vi "Dashboard Main.vi"() -> ()   [LabVIEW 2012]
uses:
  <vilib>/event_ctls.llb/eventvkey.ctl
  <vilib>/Utility/config.llb/NI_LVConfig.lvlib
  <vilib>/Utility/config.llb/Read Key (I32).vi
  <vilib>/Utility/config.llb/Write Key (I32).vi
  <vilib>/Rock Robotics/WPI/Camera/WPI_CameraExposure Priority Values.ctl
  <vilib>/Utility/config.llb/Write Key (String).vi
  <vilib>/Utility/config.llb/Read Key (String).vi
  <vilib>/Rock Robotics/WPI/Camera/WPI_CameraWhite Balance Values.ctl
panel:
  out "JS Buttons 1":cluster{bool, bool, bool, bool}={FALSE, TRUE, TRUE, FALSE}
  out "Joystick 2":cluster{"X":dbl, "Y":dbl}[](graph)
  out "Joystick 1":cluster{"X":dbl, "Y":dbl}[](graph)
  in  "STOP":bool
  in  "Camera?":bool
  in  "Brightness":i32=45
  in  "Color Level":i32=90
  in  "White Balance":T1=enum."Hold current"
  in  "Exposure Priority":T2=enum."Prioritize frame rate"
  out "Battery Value":dbl(slide) scale=0.0..14.0 scale format="%#_2e"
  out "Battery":sgl(graph)
  in  "Camera Settings":T3={"Frate Rate"=30, "Compression"=30, "Size"=1} {"Frate Rate" scale=1.0..30.0; "Size" items=["640x480", "320x240", "160x120"]}
  out "Mode":T4(ring)=enum."Auto Disabled"
  out "Robot IP":string
  in  "Dashboard Tab":enum32{"Operation", "Test", "Checklist"}(tab)
  in  "Checkbox 2":bool
  in  "Checkbox 1":bool
  in  "Slider 1":dbl(slide) scale=0.0..100.0
  in  "?":bool
  in  "Slider":dbl(slide) scale=0.0..100.0 scale format="%#_3g"
  in  "On/Off":bool caption="Solenoid"
  in  "Test Name":u16(ring) items=["Select the test to run...", "Example Test", "-------------------------------", "List of tests is built in robot code.", "Replace with your own automated tests."]
  in  "Test Tree":string(tree)
  in  "Motor":cluster{"Value":dbl, "Enable":bool} {"Value" scale=-1.0..1.0 scale format="%#_3g"}
  out "Progress":T5 {"Test Progress" scale=0.0..100.0}
  in  "Rev/Fwd":cluster{"Forward":bool, "Reverse":bool}
  in  "Ring":u16(ring) items=["Auto", "Fixed indoor", "Fixed outdoor 1", "Fixed outdoor 2", "Fixed fluorescent 1", "Fixed fluorescent 2", "Hold current"]
  in  "Listbox":i32(listbox)
  in  "Viewer":enum32{"Camera Image", "Variables"}(tab)
  out "Mbps":dbl format="%#.1g"
  in  "Enable":bool
  in  "DB Camera Config":bool
  out "Mbps":bool
  out "fps":dbl format="%#.1g"
  out "Image Error Message":string="Timeout in Camera Communications"
  out "Camera Image":T6(plugin-control)
  out "Tree":string(tree)
  # "Drive & Motors"
  # "Robot IP:"
  # "Customize by placing controls and indicators here and name to match\nDashboard Variables on robot."
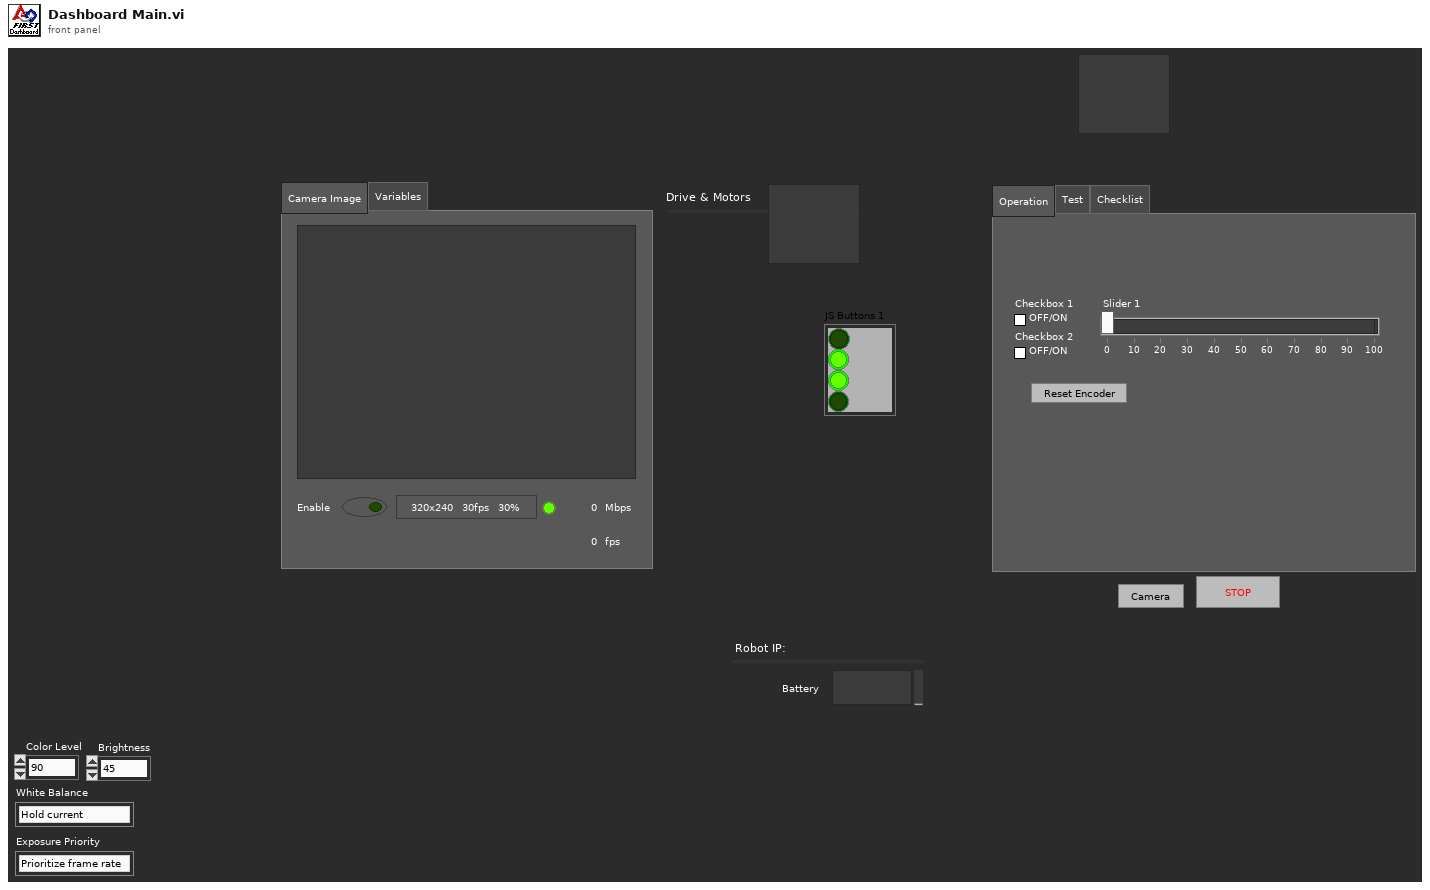
[diagram p1: front panel]
types:
  T1 = typedef "WPI_CameraWhite Balance Values.ctl" = enum16{"Auto", "Fixed indoor", "Fixed outdoor 1", "Fixed outdoor 2", "Fixed fluorescent 1", "Fixed fluorescent 2", "Hold current"}
  T2 = typedef "WPI_CameraExposure Priority Values.ctl" = enum16{"None", "Prioritize frame rate", "Prioritize image quality"}
  T3 = cluster{"Frate Rate":i32, "Compression":i32, "Size":u16}
  T4 = enum8{"Tele-Op Disabled", "Tele-Op Enabled", "Auto Disabled", "Auto Enabled", "Test Disabled", "Test Enabled", ""}
  T5 = cluster{"Test Progress":u8, "Test Progress Text":string}
  T6 = typedef "IMAQ Image.ctl" = refnum<image>
  T7 = typedef "Image Type" = u32
  T8 = cluster{"Left":i32, "Top":i32, "Right":i32, "Bottom":i32}
  T9 = typedef "WPI_CameraDevRef.ctl" = cluster{"Camera Address":string, "CameraStatus":errorcluster, "Acquire Image Notifier":refnum<notifier>}
  T10 = typedef "LVRectTypeDef.ctl" = cluster{"Left":i16, "Top":i16, "Right":i16, "Bottom":i16}
  T11 = cluster{"Competition mode":bool, "Robot Link":bool, "Autonomous":bool, "Enabled":bool, "E-Stop":bool, "Simulated":bool, "TestMode":bool, "Docked Window":bool}
  T12 = typedef "NI_LVConfig.lvlib/Config Data RefNum.ctl" = refnum<k1>
  T13 = typedef "eventvkey.ctl" = enum16{"ASCII", "Enter", "Return", "Shift", "Ctrl", "Alt", "Cmd", "Opt", "Caps", "NumLock", "Clear", "Break", "Up", "Down", "Left", "Right", "Insert", "Delete", "Home", "End", "PageUp", "PageDown", "Escape", "Help", "Pause", "ScrollLock", "F1", "F2", "F3", "F4", "F5", "F6", "F7", "F8", "F9", "F10", "F11", "F12", "F13", "F14", "F15", "F16", "F17", "F18", "F19", "F20", "F21", "F22", "F23", "F24", "Play", "VolumeUp", "VolumeDown", "Mute", "Two Byte Char"}
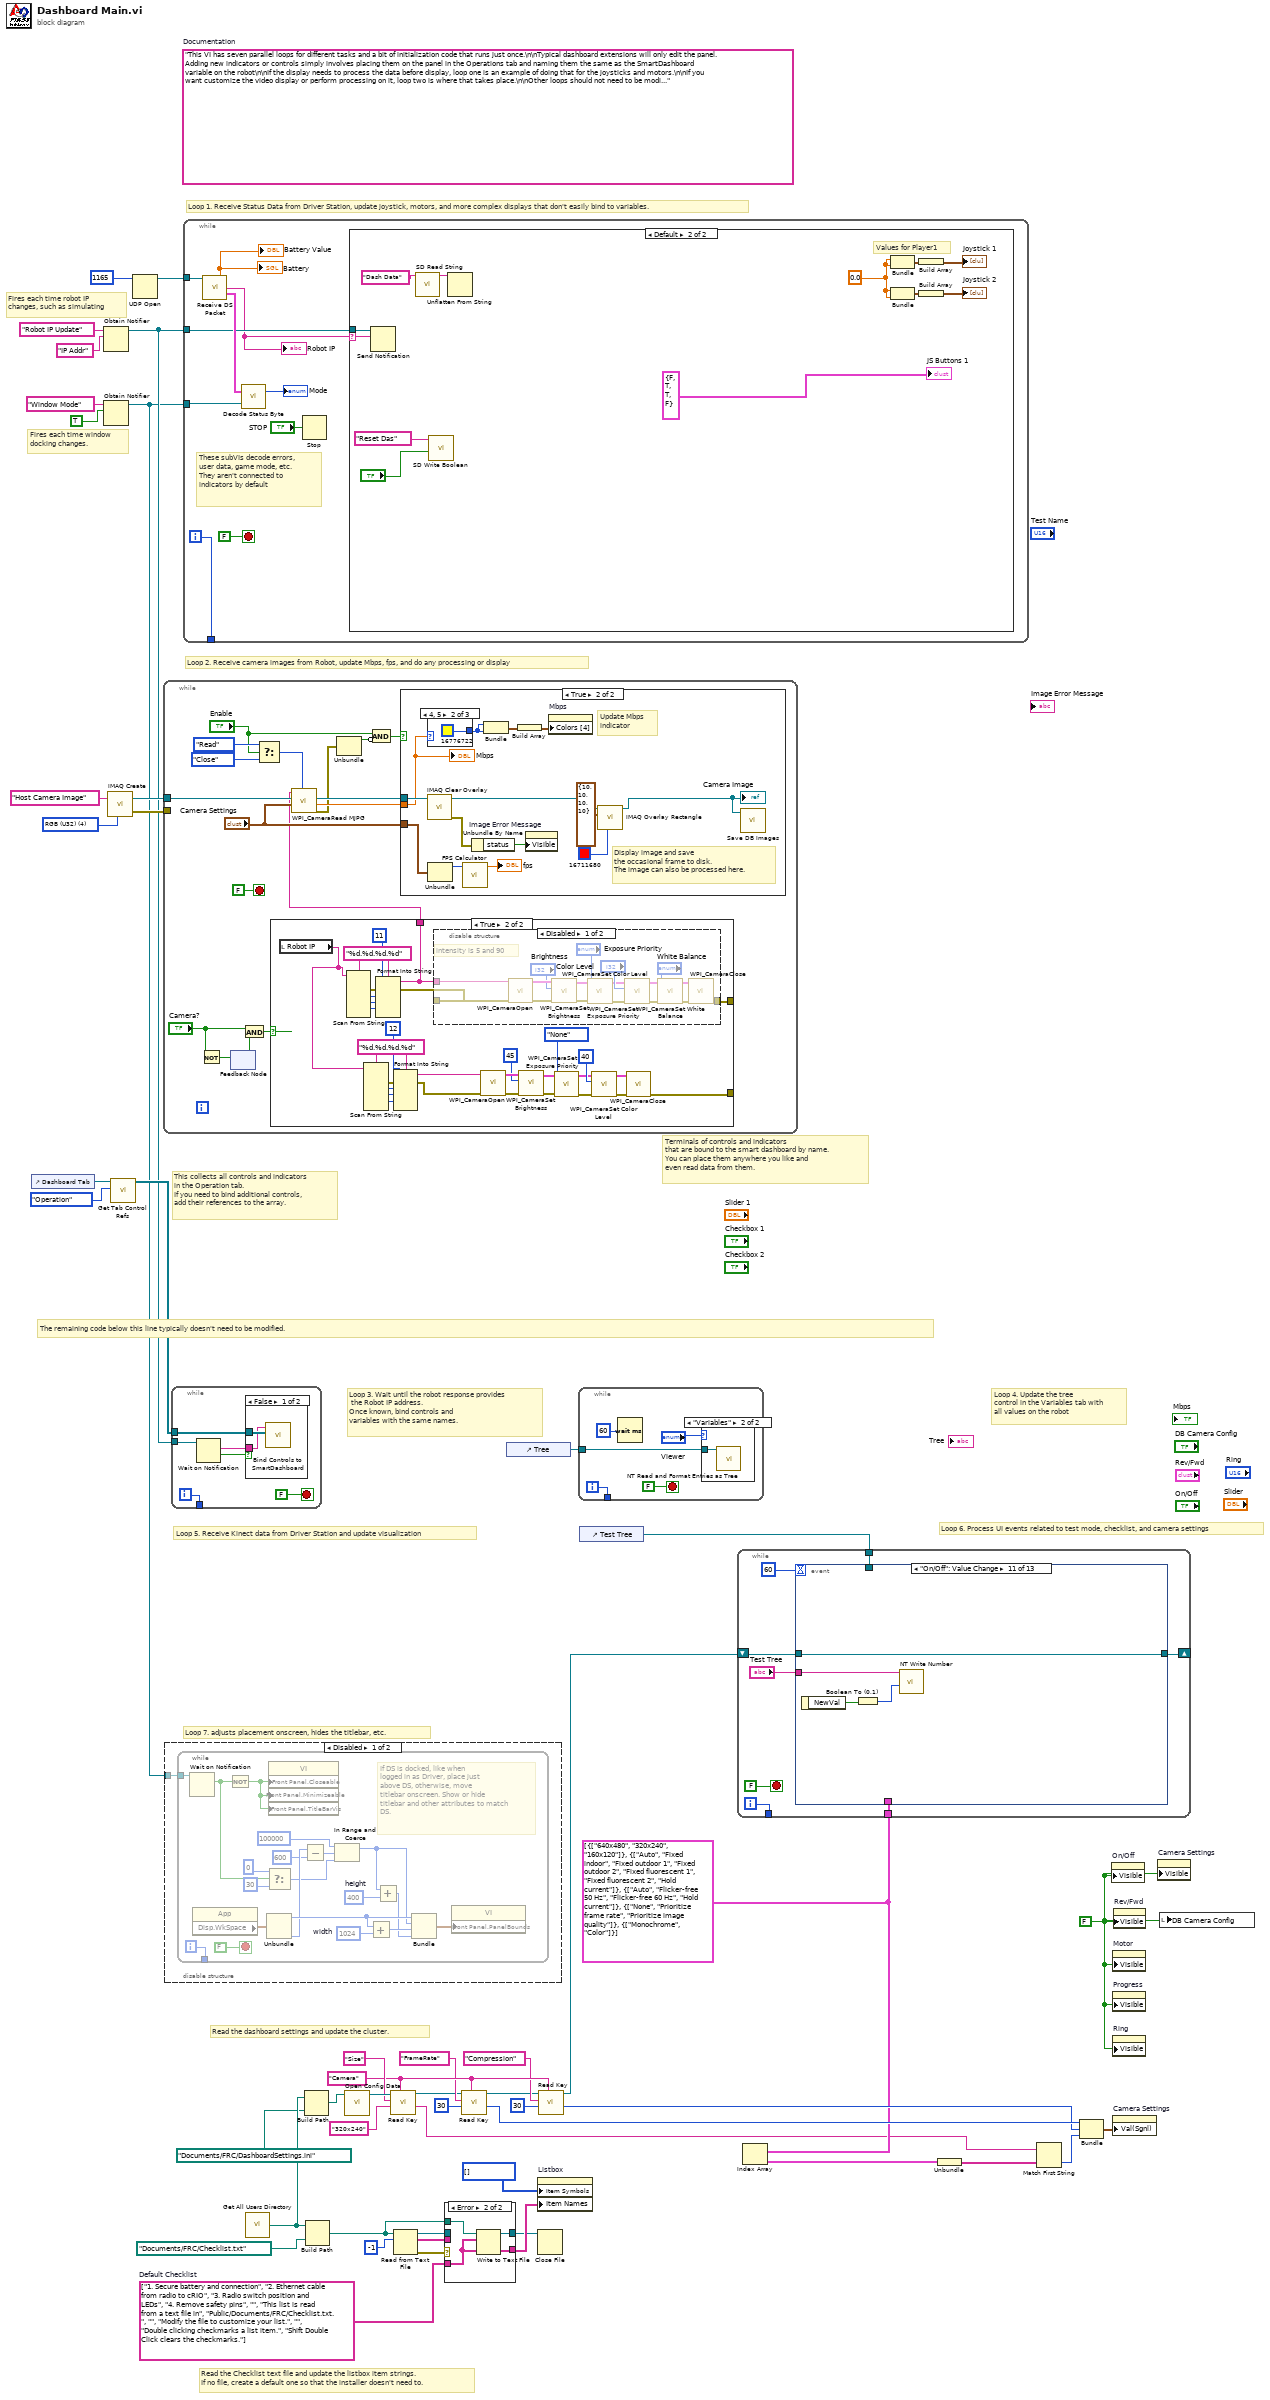
[diagram p0: block diagram]
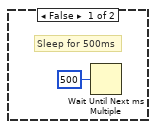
[diagram p6: hidden frame]
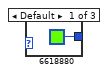
[diagram p7: hidden frame]
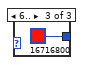
[diagram p8: hidden frame]
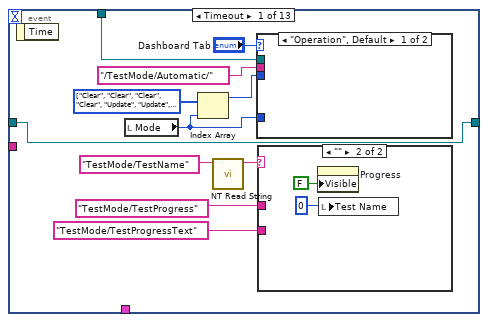
[diagram p10: hidden frame]
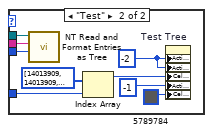
[diagram p11: hidden frame]
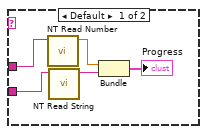
[diagram p12: hidden frame]
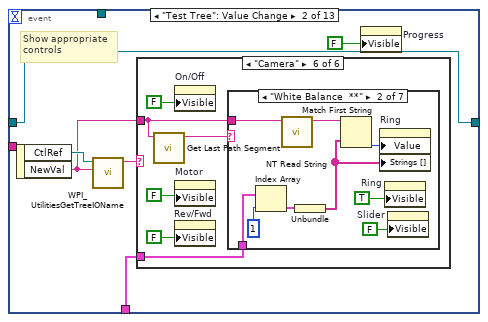
[diagram p13: hidden frame]
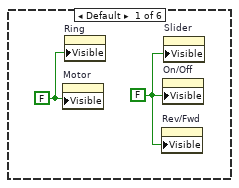
[diagram p14: hidden frame]
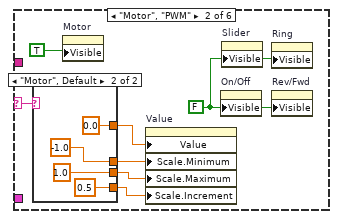
[diagram p15: hidden frame]
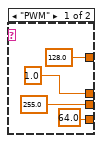
[diagram p16: hidden frame]
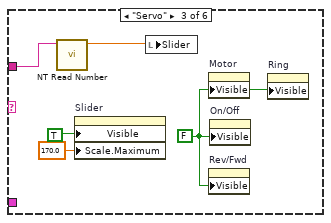
[diagram p17: hidden frame]
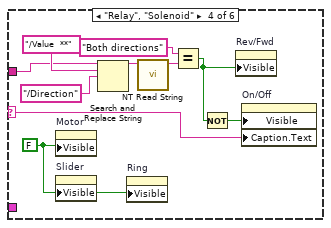
[diagram p18: hidden frame]
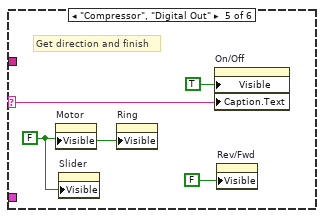
[diagram p19: hidden frame]
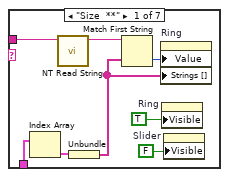
[diagram p20: hidden frame]
diagram:
  w21 = "Camera"
  w13 = cluster{string[]}[] [{["640x480", "320x240", "160x120"]}, {["Auto", "Fixed indoor", "Fixed outdoor 1", "Fixed outdoor 2", "Fixed fluorescent 1", "Fixed fluorescent 2", "Hold current"]}, {["Auto", "Flicker-free 50 Hz", "Flicker-free 60 Hz", "Hold current"]}, {["None", "Prioritize frame rate", "Prioritize image quality"]}, {["Monochrome", "Color"]}]
  w29 = string[] ["1. Secure battery and connection", "2. Ethernet cable from radio to cRIO", "3. Radio switch position and LEDs", "4. Remove safety pins", "", "This list is read from a text file in", "Public/Documents/FRC/Checklist.txt.", "", "Modify the file to customize your list.", "", "Double clicking checkmarks a list item.", "Shift Double Click clears the checkmarks."]  # Default Checklist
  w27 = FALSE ("Visible")
  (unwired) "This VI has seven parallel loops for different tasks and a bit of initialization code that runs just once.\n\nTypical dashboard extensions will only edit the panel. Adding new indicators or controls simply involves placing them on the panel in the Operations tab and naming them the same as the SmartDashboard variable on the robot\n\nIf the display needs to process the data before display, loop one is an example of doing that for the joysticks and motors.\n\nIf you want customize the video display or perform processing on it, loop two is where that takes place.\n\nOther loops should not need to be modified. They are pretty standard, and document the task they perform."  # Documentation
  w48 = T7 4 items=["Grayscale (U8)", "Grayscale (I16)", "Grayscale (SGL)", "Complex (CSG)", "RGB (U32)", "HSL (U32)", "RGB (U64)"] ("Image Type")
  # "Fires each time robot IP\nchanges, such as simulating"
  # "Fires each time window\ndocking changes."
  # "Read the Checklist text file and update the listbox item strings.\nIf no file, create a default one so that the installer doesn't need to."
  # "This collects all controls and indicators\nin the Operation tab.\nIf you need to bind additional controls,\nadd their references to the array."
  # "The remaining code below this line typically doesn't need to be modified."
  # "Loop 6. Process UI events related to test mode, checklist, and camera settings"
  # "Read the dashboard settings and update the cluster."
  # "Terminals of controls and indicators\nthat are bound to the smart dashboard by name.\nYou can place them anywhere you like and\neven read data from them."
  # "Loop 4. Update the tree\ncontrol in the Variables tab with\nall values on the robot"
  # "Loop 3. Wait until the robot response provides\n the Robot IP address.\nOnce known, bind controls and\nvariables with the same names."
  # "Loop 5. Receive Kinect data from Driver Station and update visualization"
  # "Loop 7. adjusts placement onscreen, hides the titlebar, etc."
  # "Loop 1. Receive Status Data from Driver Station, update joystick, motors, and more complex displays that don't easily bind to variables."
  # "Loop 2. Receive camera images from Robot, update Mbps, fps, and do any processing or display"
  n1 = control-ref of="Dashboard Tab"() -> (w43:refnum<vi>)
  n2 = Obtain Notifier(name (unnamed)="Robot IP Update", notification data type="IP Addr" ("name (unnamed)")) -> (notifier out=w40:refnum<notifier>)  [unwired: 2 in, 2 out]
  n3 = Obtain Notifier(name (unnamed)="Window Mode", notification data type=TRUE) -> (notifier out=w33:refnum<notifier>)  [unwired: 2 in, 2 out]
  n4 = call "IMAQ Create"("Image Name"="Host Camera Image", "Image Type"=w48) -> ("New Image"=w46:T6, "error out"=w45:errorcluster)  [unwired: 2 in, 1 out]
  n5 = call <vilib>:"Get Tab Control Refs.vi"("Page Index"=enum32{"Operation", "Test"}."Operation" ("Dashboard Tab"), "TabControl in"=w43) -> ("ControlsOnPage"=w44:refnum<vi>[])  [unwired: 9 in]
  n6 = UDP Open(11:u16 1165 ("port")) -> (port=w49:refnum<k16>)  [unwired: 2 in, 4 out]
  n7 = while {
    tunnel: w46 -> [w65]
    tunnel: w45 -> [_]
    stop <- FALSE stop-if-true
    n8 = Not(x="Camera?") -> (.not. x?=w55:bool)
    n9 = feedback #1() -> (w54:bool)  [unwired: 1 in]
    n10 = feedback-in #1(w55) -> ()
    n11 = And(x="Camera?", y=w54) -> (x .and. y?=w52:bool)
    n12 = Select(t=enum16{"Read", "Reopen", "Close"}."Read" ("Operation"), s="Enable", f=enum16{"Read", "Reopen", "Close"}."Close" ("Operation")) -> (s? t:f=w60:enum16{"Read", "Reopen", "Close"})
    n13 = case shown="True" w52 {
      tunnel: [_ w90] -> _
      tunnel: [_ w70] -> _
      tunnel: [_ w68] -> w51
      frame False {
      }
      frame True {
        w77 = "%d.%d.%d.%d" ("format string")
        w92 = "%d.%d.%d.%d" ("format string")
        n14 = local read "Robot IP"() -> (w69:string)
        n15 = Scan From String(format string=w92, input string=w69) -> (error out=w94:errorcluster, output 1=w95:i32, output 2=w96:i32, output 3=w97:i32)  [unwired: 2 in, 7 out]
        n16 = Scan From String(format string=w77, input string=w69) -> (error out=w79:errorcluster, output 1=w80:i32, output 2=w81:i32, output 3=w82:i32)  [unwired: 2 in, 7 out]
        n17 = Format Into String(format string=w92, error in=w94, w95, w96, w97, 11 ("IP Suffix:")) -> (resulting string=w68:string, error out=w91:errorcluster)  [unwired: 1 in]
        n18 = Format Into String(format string=w77, error in=w79, w80, w81, w82, 12 ("IP Suffix:")) -> (resulting string=w71:string, error out=w72:errorcluster)  [unwired: 1 in]
        n19 = disable-structure shown="Disabled" {
          disable-tunnel: w91 -> [w106 _]
          disable-tunnel: w68 -> [w105 _]
          disable-tunnel: [w104 _] -> w90
          frame Disabled {
            # "intensity is 5 and 90"
            n20 = call <vilib>:"WPI_CameraOpen.vi"("error in (no error)"=w106, "Camera Address"=w105) -> ("error out"=w109:errorcluster, "CameraDevRef"=w111:T9)  [unwired: 8 in]
            n21 = call <vilib>:"WPI_CameraSet Brightness.vi"("error in (no error)"=w109, "Brightness"="Brightness", "CameraDevRef"=w111) -> ("error out"=w108:errorcluster, "CameraDevRef Out"=w98:T9)  [unwired: 7 in]
            n22 = call <vilib>:"WPI_CameraSet Exposure Priority.vi"("error in (no error)"=w108, "Exposure Priority"="Exposure Priority", "CameraDevRef"=w98) -> ("error out"=w107:errorcluster, "CameraDevRef Out"=w113:T9)  [unwired: 7 in]
            n23 = call <vilib>:"WPI_CameraSet Color Level.vi"("error in (no error)"=w107, "Color Level"="Color Level", "CameraDevRef"=w113) -> ("error out"=w100:errorcluster, "CameraDevRef Out"=w101:T9)  [unwired: 7 in]
            n24 = call <vilib>:"WPI_CameraSet White Balance.vi"("error in (no error)"=w100, "White Balance"="White Balance", "CameraDevRef"=w101) -> ("error out"=w99:errorcluster, "CameraDevRef Out"=w102:T9)  [unwired: 7 in]
            n25 = call <vilib>:"WPI_CameraClose.vi"("error in (no error)"=w99, "CameraDevRef"=w102) -> ("error out"=w104:errorcluster)  [unwired: 9 in]
          }
          frame Enabled {
          }
        }
        n26 = call <vilib>:"WPI_CameraOpen.vi"("error in (no error)"=w72, "Camera Address"=w71) -> ("error out"=w76:errorcluster, "CameraDevRef"=w84:T9)  [unwired: 8 in]
        n27 = call <vilib>:"WPI_CameraSet Brightness.vi"("error in (no error)"=w76, "Brightness"=45, "CameraDevRef"=w84) -> ("error out"=w75:errorcluster, "CameraDevRef Out"=w85:T9)  [unwired: 7 in]
        n28 = call <vilib>:"WPI_CameraSet Exposure Priority.vi"("error in (no error)"=w75, "Exposure Priority"=WPI_CameraExposure_Priority_Values."None", "CameraDevRef"=w85) -> ("error out"=w74:errorcluster, "CameraDevRef Out"=w88:T9)  [unwired: 7 in]
        n29 = call <vilib>:"WPI_CameraSet Color Level.vi"("error in (no error)"=w74, "Color Level"=40, "CameraDevRef"=w88) -> ("error out"=w73:errorcluster, "CameraDevRef Out"=w87:T9)  [unwired: 7 in]
        n30 = call <vilib>:"WPI_CameraClose.vi"("error in (no error)"=w73, "CameraDevRef"=w87) -> ("error out"=w70:errorcluster)  [unwired: 9 in]
      }
    }
    n31 = call <vilib>:"WPI_CameraRead MJPG.vi"("Operation"=w60, "Camera Settings"="Camera Settings", "Image"=w65, "address"=w51) -> ("error out"=w59:errorcluster, "Bandwidth (kbps)"=w63:dbl, "Image Out"=w64:T6)  [unwired: 5 in]
    n32 = Unbundle(w59) -> ("status"=w57:bool)  [unwired: 2 out]
    n33 = Compound Arithmetic op=AND("Enable", invert w57) -> (w56:bool)
    n34 = case shown="True" w56 {
      tunnel: "Camera Settings" -> [_ w121]
      tunnel: w64 -> [_ w124]
      tunnel: w63 -> [_ w123]
      frame False {
        # "Sleep for 500ms"
        n35 = Wait Until Next ms Multiple(millisecond multiple=u32 500) -> ()  [unwired: 1 out]
      }
      frame True {
        # "Display image and save\nthe occasional frame to disk.\nThe image can also be processed here."
        # "Update Mbps\nindicator"
        n36 = call "IMAQ Clear Overlay"("Image"=w124) -> ("error out"=w128:errorcluster, "Image Out"=w119:T6)  [unwired: 2 in, 7 out]
        n37 = case shown="4, 5" w123 {
          tunnel: [u32 6618880 ("Color Box") u32 16776722 ("Color Box") u32 16716800 ("Color Box")] -> w125
          frame Default {
          }
          frame 4, 5 {
          }
          frame 6.. {
          }
        }
        n38 = Unbundle(w121) -> ("Frate Rate"=w120:i32)  [unwired: 2 out]
        n39 = call "FPS Calculator.vi"("Average Count"=w120) -> ("fps"=→"fps":dbl)  [unwired: 10 in]
        n40 = Unbundle By Name(w128) -> ("status"=w129:bool)
        n41 = Bundle("Color Box"=w125, "Color Box"=w125) -> (w127:cluster{"Color Box":u32, "Color Box":u32})  [unwired: 1 out]
        n42 = Build Array(w127) -> (w126:cluster{"Color Box":u32, "Color Box":u32}[])
        n43 = property on="Image Error Message" class="Str"("Visible"=w129) -> ()  [unwired: 2 in, 2 out]
        n44 = property on="Mbps" class="Bool (strict)"("Colors [4]"=w126) -> ()  [unwired: 2 in, 2 out]
        n45 = call "IMAQ Overlay Rectangle"("Color"=u32 16711680, "Rectangle"=T8 {"Left"=10, "Top"=10, "Right"=10, "Bottom"=10}, "Image"=w119) -> ("Image Out"=w118:T6)  [unwired: 7 in, 1 out]
        "Camera Image" <- w118
        n46 = call "Save DB Images.vi"("Image"=w118) -> ()  [unwired: 2 in, 1 out]
        "Mbps" <- w123
      }
    }
  }
  n47 = disable-structure shown="Disabled" {
    disable-tunnel: w33 -> [w133 _]
    frame Disabled {
      n48 = while {
        tunnel: w133 -> [w152]
        tunnel: [w150] -> _
        i -> [w150]
        stop <- FALSE stop-if-true
        w142 = 1024  # width
        w145 = 400  # height
        # "If DS is docked, like when\nlogged in as Driver, place just\nabove DS, otherwise, move\ntitlebar onscreen. Show or hide\ntitlebar and other attributes to match\nDS."
        n49 = Wait on Notification(notifier=w152) -> (notification=w137:bool)  [unwired: 3 in, 3 out]
        n50 = property class="App"() -> ("Disp.WkSpace"=w148:T10)  [unwired: 2 in, 2 out]
        n51 = Not(x=w137) -> (.not. x?=w151:bool)
        n52 = Unbundle(w148) -> ("Left"=w146:i16, "Bottom"=w143:i16)  [unwired: 2 out]
        n53 = Select(t=0, s=w137, f=30) -> (s? t:f=w136:i32)
        n54 = property class="VI"("Front Panel.Closeable"=w151, "Front Panel.Minimizeable"=w151, "Front Panel.TitleBarVis"=w151) -> ()  [unwired: 2 in, 2 out]
        n55 = Subtract(x=w143, y=600) -> (x-y=w140:i32)
        n56 = In Range and Coerce(upper limit=100000, x=w140, lower limit=w136) -> (coerced(x)=w134:i32)  [unwired: 1 out]
        n57 = Add(x=w146, y=w142) -> (x+y=w147:i32)
        n58 = Add(x=w134, y=w145) -> (x+y=w144:i32)
        n59 = Bundle("Left"=w146, w134, w147, w144) -> (w149:cluster{"Left":i16, i32, i32, i32})  [unwired: 1 out]
        n60 = property class="VI"("Front Panel.PanelBounds"=w149) -> ()  [unwired: 2 in, 2 out]
      }
    }
    frame Enabled {
    }
  }
  n61 = while {
    tunnel: w44 -> [w159]
    tunnel: w40 -> [w156]
    tunnel: [w154] -> _
    i -> [w154]
    stop <- FALSE stop-if-true
    n62 = Wait on Notification(notifier=w156) -> (notification=w155:string, timed out?=w157:bool)  [unwired: 3 in, 2 out]
    n63 = case shown="False" w157 {
      tunnel: w159 -> [w161 _]
      tunnel: w155 -> [w160 _]
      frame False {
        n64 = call <vilib>:"Bind Controls to SmartDashboard.vi"("Bound Control Refs"=w161, "Server IP Address"=w160) -> ()  [unwired: 10 in]
      }
      frame True {
      }
    }
  }
  n65 = while {
    tunnel: w49 -> [w169]
    tunnel: w40 -> [w164]
    tunnel: w33 -> [w167]
    tunnel: [w165] -> _
    i -> [w165]
    stop <- FALSE stop-if-true
    # "These subVIs decode errors, user data, game mode, etc.\nThey aren't connected to indicators by default"
    n66 = call "Receive DS Packet.vi"("Recv Socket"=w169) -> ("Battery"=→"Battery" →"Battery Value":sgl, "Robot IP Address"=w163:string, "Status"=w170:T11)  [unwired: 1 in, 11 out]
    "Robot IP" <- w163
    n67 = call "Decode Status Byte.vi"("Window Mode Notifier"=w167, "Status"=w170) -> ("Mode"=→"Mode":T4)  [unwired: 1 out]
    n68 = Stop(stop? (T)="STOP") -> ()
    n69 = case shown="Default" w163 {
      selector: w163 -> [_ w182]
      tunnel: w164 -> [_ w183]
      frame "0.0.0.0" {
        # "Robot not responding, don't poll the variables"
      }
      frame Default {
        w173 = 0.0
        # "Values for Player1"
        n70 = Send Notification(notification=w182, notifier=w183) -> ()  [unwired: 1 in, 2 out]
        n71 = call <vilib>:"SD Read String.vi"("Name"="Dash Data") -> ("String"=w180:string)  [unwired: 8 in, 2 out]
        n72 = call <vilib>:"SD Write Boolean.vi"("Boolean"="?", "Name"="Reset Das") -> ()  [unwired: 8 in, 2 out]
        n73 = Unflatten From String(binary string=w180) -> ()  [unwired: 4 in, 3 out]
        n74 = Bundle(w173, w173) -> (w177:cluster{dbl, dbl})  [unwired: 1 in]
        n75 = Bundle(w173, w173) -> (w175:cluster{dbl, dbl})  [unwired: 1 in]
        n76 = Build Array(w177) -> (→"Joystick 1":cluster{dbl, dbl}[])
        n77 = Build Array(w175) -> (→"Joystick 2":cluster{dbl, dbl}[])
        "JS Buttons 1" <- cluster{bool, bool, bool, bool} {FALSE, TRUE, TRUE, FALSE} ("JS Buttons 1")
      }
    }
  }
  n78 = call "Get All Users Directory.vi"() -> ("All User Path"=w26:path)
  n79 = Build Path(base path=w26, name or relative path=path "Documents/FRC/DashboardSettings.ini") -> (appended path=w25:path)
  n80 = Build Path(base path=w26, name or relative path=path "Documents/FRC/Checklist.txt") -> (appended path=w30:path)
  n81 = call <vilib>:"Open Config Data.vi"("configuration file path"=w25) -> ("refnum"=w24:T12)  [unwired: 8 in, 2 out]
  n82 = call-poly <vilib>:"Read Key.vi"("section"=w21, "default value"="320x240", "key"="Size", "refnum"=w24) -> ("value"=w11:string, "refnum out"=w6:T12)  [unwired: 2 in, 4 out]
  n83 = Read from Text File(file (use dialog)=w30, count=-1 ("timeout ms (25000)")) -> (refnum out=w8:refnum<file>, text=w31:string[], error out=w32:errorcluster)  [unwired: 2 in, 1 out]
  n84 = case shown="Error" w32 {
    tunnel: w31 -> [w185 _]
    tunnel: [w185 w187] -> w28
    tunnel: w29 -> [_ w187]
    tunnel: w30 -> [_ w188]
    tunnel: [w184 w186] -> w7
    tunnel: w8 -> [w184 _]
    frame No Error {
    }
    frame Error {
      n85 = Write to Text File(file (use dialog)=w188, text=w187) -> (refnum out=w186:refnum<file>)  [unwired: 2 in, 2 out]
    }
  }
  n86 = call-poly <vilib>:"Read Key.vi"("section"=w21, "default value"=30, "key"="FrameRate", "refnum"=w6) -> ("value"=w16:i32, "refnum out"=w5:T12)  [unwired: 1 in, 5 out]
  n87 = control-ref of="Tree"() -> (w2:refnum<vi>)
  n88 = property on="Listbox" class="LstBox (strict)"("Item Symbols"=i32[] [], "Item Names"=w28) -> ()  [unwired: 2 in, 2 out]
  n89 = Close File(refnum=w7) -> ()  [unwired: 1 in, 2 out]
  n90 = call-poly <vilib>:"Read Key.vi"("section"=w21, "default value"=30, "key"="Compression", "refnum"=w5) -> ("value"=w15:i32, "refnum out"=w3:T12)  [unwired: 1 in, 5 out]
  n91 = while {
    tunnel: [w190] -> _
    tunnel: w2 -> [w189]
    i -> [w190]
    stop <- FALSE stop-if-true
    n92 = Wait (ms)(milliseconds to wait=u32 60) -> ()  [unwired: 1 out]
    n93 = case shown="\"Variables\"" "Viewer" {
      tunnel: w189 -> [_ w194]
      frame Default {
      }
      frame "Variables" {
        n94 = call <vilib>:"NT Read and Format Entries as Tree.vi"("Tree Refnum"=w194) -> ()  [unwired: 9 in, 2 out]
      }
    }
  }
  n95 = control-ref of="Test Tree"() -> (w1:refnum<vi>)
  n96 = while {
    tunnel: w13 -> [w199]
    shift-right: [w198] -> _
    shift-left: w3 -> [w197]
    tunnel: [w196] -> _
    tunnel: w1 -> [w195]
    i -> [w196]
    stop <- FALSE stop-if-true
    n97 = event shown="[10] \"On/Off \": Value Change" {
      selector: _ -> [_ _ _ _ _ _ _ _ _ _ _ _ _]
      dyn-events: _ -> [_ _ _ _ _ _ _ _ _ _ _ _ _]
      timeout: u32 60 ("milliseconds to wait") -> [_ _ _ _ _ _ _ _ _ _ _ _ _]
      tunnel: w195 -> [w209 _ _ _ _ _ _ _ _ _ _ _ _]
      tunnel: "Test Tree" -> [_ _ _ _ _ _ _ _ w403 w411 w413 w417 w425]
      tunnel: w199 -> [_ w231 _ _ _ _ w367 w397 _ _ _ _ _]
      tunnel: [w203 w230 _ w333 w341 w353 w366 w390 w402 w409 w412 w416 w424] -> w198
      tunnel: w197 -> [w203 w230 _ w333 w341 w353 w365 w390 w402 w409 w412 w416 w424]
      event Timeout {
        w208 = enum16{"Update", "Clear"}[] [enum."Clear", enum."Clear", enum."Clear", enum."Clear", enum."Update", enum."Update", enum."Clear"] items=["Update", "Clear"]
        n98 = event-data() -> ()  [unwired: 1 in, 1 out]
        n99 = local read "Mode"() -> (w206:T4)
        n100 = Index Array(array=w208, index=w206) -> (element=w207:enum16{"Update", "Clear"})
        n101 = call <vilib>:"NT Read String.vi"("Name"="TestMode/TestName") -> ("String"=w212:string)  [unwired: 9 in, 1 out]
        n102 = case shown="\"Operation\", Default" "Dashboard Tab" {
          tunnel: w209 -> [_ w222]
          tunnel: "/TestMode/Automatic/" ("Name Pattern") -> [_ w221]
          tunnel: w207 -> [_ w220]
          tunnel: w206 -> [_ w218]
          frame "Operation", Default {
          }
          frame "Test" {
            w217 = -2 ("Active Item:Row Number")
            n103 = call <vilib>:"NT Read and Format Entries as Tree.vi"("Operation"=w220, "Name Pattern"=w221, "Tree Refnum"=w222) -> ()  [unwired: 7 in, 2 out]
            n104 = Index Array(array=u32[] [14013909, 14013909, 14013909, 14013909, 14013909, 16777215, 14013909], index=w218) -> (element=w216:u32)
            n105 = property on="Test Tree" class="Tree (strict)"("Active Item Row Number"=w217, "ActiveColNum"=w217, "CellBG"=w216, "Active Item Row Number"=-1 ("Active Item:Row Number"), "CellBG"=u32 5789784 ("Color Box")) -> ()  [unwired: 2 in, 2 out]
          }
        }
        n106 = case shown="\"\"" w212 {
          tunnel: "TestMode/TestProgress" ("Name") -> [w224 _]
          tunnel: "TestMode/TestProgressText" ("Name") -> [w223 _]
          frame Default {
            n107 = call <vilib>:"NT Read Number.vi"("Name"=w224) -> ("Numeric"=w225:dbl)  [unwired: 9 in, 1 out]
            n108 = call <vilib>:"NT Read String.vi"("Name"=w223) -> ("String"=w226:string)  [unwired: 9 in, 1 out]
            n109 = Bundle("Numeric"=w225, "String"=w226) -> (→"Progress":cluster{"Numeric":dbl, "String":string})  [unwired: 1 in]
          }
          frame "" {
            n110 = property on="Progress" class="Clust (strict)"("Visible"=FALSE) -> ()  [unwired: 2 in, 2 out]
            n111 = local write "Test Name"(u16 0) -> ()
          }
        }
      }
      event "Test Tree": Value Change {
        # "Show appropriate\ncontrols"
        n112 = event-data() -> ("CtlRef"=w234:refnum<vi>, "NewVal"=w232:string)  [unwired: 1 in]
        n113 = call <vilib>:"WPI_UtilitiesGetTreeIOName.vi"("NewVal"=w232, "TreeControl in"=w234) -> ("I/O Name"=w235:string)  [unwired: 9 in]
        n114 = case shown="\"Camera\"" w235 {
          selector: w235 -> [_ w242 _ w260 w269 _]
          tunnel: w232 -> [_ _ w257 w259 _ w276]
          tunnel: w231 -> [_ _ _ _ _ w275]
          frame Default {
            w237 = FALSE ("Visible")
            w236 = FALSE ("Visible")
            n115 = property on="Motor" class="Clust (strict)"("Visible"=w236) -> ()  [unwired: 2 in, 2 out]
            n116 = property on="Ring" class="Ring (strict)"("Visible"=w236) -> ()  [unwired: 2 in, 2 out]
            n117 = property on="Rev/Fwd" class="Clust (strict)"("Visible"=w237) -> ()  [unwired: 2 in, 2 out]
            n118 = property on="On/Off" class="Bool (strict)"("Visible"=w237) -> ()  [unwired: 2 in, 2 out]
            n119 = property on="Slider" class="Slide (strict)"("Visible"=w237) -> ()  [unwired: 2 in, 2 out]
          }
          frame "Motor", "PWM" {
            w243 = FALSE ("Visible")
            n120 = case shown="\"Motor\", Default" w242 {
              tunnel: [1.0 ("Value") -1.0 ("Value")] -> w241
              tunnel: [255.0 ("Value") 1.0 ("Value")] -> w240
              tunnel: [128.0 ("Value") 0.0 ("Value")] -> w239
              tunnel: [64.0 ("Value") 0.5 ("Value")] -> w238
              frame "PWM" {
              }
              frame "Motor", Default {
              }
            }
            n121 = property on="Motor" class="Clust (strict)"("Visible"=TRUE) -> ()  [unwired: 2 in, 2 out]
            n122 = property on="Value" class="Slide (strict)"("Value"=w239, "Scale.Minimum"=w241, "Scale.Maximum"=w240, "Scale.Increment"=w238) -> ()  [unwired: 2 in, 2 out]
            n123 = property on="On/Off" class="Bool (strict)"("Visible"=w243) -> ()  [unwired: 2 in, 2 out]
            n124 = property on="Slider" class="Slide (strict)"("Visible"=w243) -> ()  [unwired: 2 in, 2 out]
            n125 = property on="Ring" class="Ring (strict)"("Visible"=w243) -> ()  [unwired: 2 in, 2 out]
            n126 = property on="Rev/Fwd" class="Clust (strict)"("Visible"=w243) -> ()  [unwired: 2 in, 2 out]
          }
          frame "Servo" {
            w255 = FALSE ("Visible")
            n127 = call <vilib>:"NT Read Number.vi"("Name"=w257) -> ("Numeric"=w256:dbl)  [unwired: 9 in, 1 out]
            n128 = property on="Slider" class="Slide (strict)"("Visible"=TRUE, "Scale.Maximum"=170.0 ("Scale.Range:Maximum")) -> ()  [unwired: 2 in, 2 out]
            n129 = local write "Slider"(w256) -> ()
            n130 = property on="Motor" class="Clust (strict)"("Visible"=w255) -> ()  [unwired: 2 in, 2 out]
            n131 = property on="Rev/Fwd" class="Clust (strict)"("Visible"=w255) -> ()  [unwired: 2 in, 2 out]
            n132 = property on="On/Off" class="Bool (strict)"("Visible"=w255) -> ()  [unwired: 2 in, 2 out]
            n133 = property on="Ring" class="Ring (strict)"("Visible"=w255) -> ()  [unwired: 2 in, 2 out]
          }
          frame "Relay", "Solenoid" {
            w258 = FALSE ("Visible")
            n134 = property on="Motor" class="Clust (strict)"("Visible"=w258) -> ()  [unwired: 2 in, 2 out]
            n135 = property on="Slider" class="Slide (strict)"("Visible"=w258) -> ()  [unwired: 2 in, 2 out]
            n136 = Search and Replace String(input string=w259, search string="/Value  **", replace string="/Direction") -> (result string=w265:string)  [unwired: 5 in, 3 out]
            n137 = property on="Ring" class="Ring (strict)"("Visible"=w258) -> ()  [unwired: 2 in, 2 out]
            n138 = call <vilib>:"NT Read String.vi"("Name"=w265) -> ("String"=w263:string)  [unwired: 9 in, 1 out]
            n139 = Equal?(x="Both directions", y=w263) -> (x = y?=w261:bool)
            n140 = Not(x=w261) -> (.not. x?=w262:bool)
            n141 = property on="Rev/Fwd" class="Clust (strict)"("Visible"=w261) -> ()  [unwired: 2 in, 2 out]
            n142 = property on="On/Off" class="Bool (strict)"("Visible"=w262, "Caption.Text"=w260) -> ()  [unwired: 2 in, 2 out]
          }
          frame "Compressor", "Digital Out" {
            w268 = FALSE ("Visible")
            # "Get direction and finish"
            n143 = property on="Motor" class="Clust (strict)"("Visible"=w268) -> ()  [unwired: 2 in, 2 out]
            n144 = property on="Slider" class="Slide (strict)"("Visible"=w268) -> ()  [unwired: 2 in, 2 out]
            n145 = property on="Ring" class="Ring (strict)"("Visible"=w268) -> ()  [unwired: 2 in, 2 out]
            n146 = property on="On/Off" class="Bool (strict)"("Visible"=TRUE, "Caption.Text"=w269) -> ()  [unwired: 2 in, 2 out]
            n147 = property on="Rev/Fwd" class="Clust (strict)"("Visible"=FALSE) -> ()  [unwired: 2 in, 2 out]
          }
          frame "Camera" {
            n148 = call <vilib>:"Get Last Path Segment.vi"("String in"=w276) -> ("String out"=w277:string)  [unwired: 10 in]
            n149 = property on="On/Off" class="Bool (strict)"("Visible"=FALSE) -> ()  [unwired: 2 in, 2 out]
            n150 = property on="Motor" class="Clust (strict)"("Visible"=FALSE) -> ()  [unwired: 2 in, 2 out]
            n151 = property on="Rev/Fwd" class="Clust (strict)"("Visible"=FALSE) -> ()  [unwired: 2 in, 2 out]
            n152 = case shown="\"White Balance  **\"" w277 {
              tunnel: w276 -> [w283 w292 w301 w310 w319 _ w325]
              tunnel: w275 -> [w281 w289 w298 w307 w316 _ _]
              frame "Size  **" {
                n153 = Index Array(array=w281) -> (element=w280:cluster{string[]})  [unwired: 1 in]
                n154 = call <vilib>:"NT Read String.vi"("Name"=w283) -> ("String"=w282:string)  [unwired: 9 in, 1 out]
                n155 = Unbundle(w280) -> (w278:string[])
                n156 = Match First String(2:w278, 3:w282) -> (0:w279:i32)  [unwired: 1 out]
                n157 = property on="Ring" class="Ring (strict)"("Value"=w279, "Strings []"=w278) -> ()  [unwired: 2 in, 2 out]
                n158 = property on="Ring" class="Ring (strict)"("Visible"=TRUE) -> ()  [unwired: 2 in, 2 out]
                n159 = property on="Slider" class="Slide (strict)"("Visible"=FALSE) -> ()  [unwired: 2 in, 2 out]
              }
              frame "White Balance  **" {
                n160 = Index Array(array=w289, index=1) -> (element=w290:cluster{string[]})
                n161 = call <vilib>:"NT Read String.vi"("Name"=w292) -> ("String"=w291:string)  [unwired: 9 in, 1 out]
                n162 = Unbundle(w290) -> (w287:string[])
                n163 = Match First String(2:w287, 3:w291) -> (0:w286:i32)  [unwired: 1 out]
                n164 = property on="Ring" class="Ring (strict)"("Value"=w286, "Strings []"=w287) -> ()  [unwired: 2 in, 2 out]
                n165 = property on="Ring" class="Ring (strict)"("Visible"=TRUE) -> ()  [unwired: 2 in, 2 out]
                n166 = property on="Slider" class="Slide (strict)"("Visible"=FALSE) -> ()  [unwired: 2 in, 2 out]
              }
              frame "Exposure  **" {
                n167 = Index Array(array=w298, index=2) -> (element=w299:cluster{string[]})
                n168 = call <vilib>:"NT Read String.vi"("Name"=w301) -> ("String"=w300:string)  [unwired: 9 in, 1 out]
                n169 = Unbundle(w299) -> (w295:string[])
                n170 = Match First String(2:w295, 3:w300) -> (0:w296:i32)  [unwired: 1 out]
                n171 = property on="Ring" class="Ring (strict)"("Value"=w296, "Strings []"=w295) -> ()  [unwired: 2 in, 2 out]
                n172 = property on="Ring" class="Ring (strict)"("Visible"=TRUE) -> ()  [unwired: 2 in, 2 out]
                n173 = property on="Slider" class="Slide (strict)"("Visible"=FALSE) -> ()  [unwired: 2 in, 2 out]
              }
              frame "Exposure Priority  **" {
                n174 = Index Array(array=w307, index=3) -> (element=w308:cluster{string[]})
                n175 = call <vilib>:"NT Read String.vi"("Name"=w310) -> ("String"=w309:string)  [unwired: 9 in, 1 out]
                n176 = Unbundle(w308) -> (w304:string[])
                n177 = Match First String(2:w304, 3:w309) -> (0:w305:i32)  [unwired: 1 out]
                n178 = property on="Ring" class="Ring (strict)"("Value"=w305, "Strings []"=w304) -> ()  [unwired: 2 in, 2 out]
                n179 = property on="Ring" class="Ring (strict)"("Visible"=TRUE) -> ()  [unwired: 2 in, 2 out]
                n180 = property on="Slider" class="Slide (strict)"("Visible"=FALSE) -> ()  [unwired: 2 in, 2 out]
              }
              frame "Color Enable  **" {
                n181 = Index Array(array=w316, index=4) -> (element=w317:cluster{string[]})
                n182 = call <vilib>:"NT Read String.vi"("Name"=w319) -> ("String"=w318:string)  [unwired: 9 in, 1 out]
                n183 = Unbundle(w317) -> (w313:string[])
                n184 = Match First String(2:w313, 3:w318) -> (0:w314:i32)  [unwired: 1 out]
                n185 = property on="Ring" class="Ring (strict)"("Value"=w314, "Strings []"=w313) -> ()  [unwired: 2 in, 2 out]
                n186 = property on="Ring" class="Ring (strict)"("Visible"=TRUE) -> ()  [unwired: 2 in, 2 out]
                n187 = property on="Slider" class="Slide (strict)"("Visible"=FALSE) -> ()  [unwired: 2 in, 2 out]
              }
              frame Default {
                n188 = property on="Ring" class="Ring (strict)"("Visible"=FALSE) -> ()  [unwired: 2 in, 2 out]
                n189 = property on="Slider" class="Slide (strict)"("Visible"=FALSE) -> ()  [unwired: 2 in, 2 out]
              }
              frame "Brightness  **", "Color Level  **", "Compression  **", "FPS  **", "Sharpness  **" {
                n190 = call <vilib>:"NT Read Number.vi"("Name"=w325) -> ("Numeric"=w324:dbl)  [unwired: 9 in, 1 out]
                n191 = local write "Slider"(w324) -> ()
                n192 = property on="Slider" class="Slide (strict)"("Visible"=TRUE, "Scale.Maximum"=100.0 ("Scale.Range:Maximum")) -> ()  [unwired: 2 in, 2 out]
                n193 = property on="Ring" class="Ring (strict)"("Visible"=FALSE) -> ()  [unwired: 2 in, 2 out]
              }
            }
          }
        }
        n194 = property on="Progress" class="Clust (strict)"("Visible"=FALSE) -> ()  [unwired: 2 in, 2 out]
      }
      event "Test Name": Mouse Enter {
        # "Populate the ring with the list of tests"
        n195 = event-data() -> ()  [unwired: 1 in, 1 out]
        n196 = call <vilib>:"NT Read String Array.vi"("Name"="TestMode/TestList") -> ("String Array"=w332:string[])  [unwired: 9 in, 1 out]
        n197 = Build Array (concatenate)("Select the test to run...", w332) -> (w331:string[])
        n198 = property on="Test Name" class="Ring (strict)"("Strings []"=w331) -> ()  [unwired: 2 in, 2 out]
      }
      event "Test Name": Value Change {
        w334 = FALSE ("Visible")
        # "Tell the robot the test name to run"
        n199 = event-data() -> ("NewVal"=w338:u16)  [unwired: 1 in]
        n200 = property on="Test Name" class="Ring (strict)"() -> ("Strings []"=w339:string[])  [unwired: 2 in, 2 out]
        n201 = local write "Progress"(T5 {"Test Progress"=0, "Test Progress Text"=""} ("Progress")) -> ()
        n202 = Index Array(array=w339, index=w338) -> (element=w337:string)
        n203 = call <vilib>:"NT Write String.vi"("String"=w337, "Name"="TestMode/TestName") -> ()  [unwired: 9 in, 1 out]
        n204 = property on="Progress" class="Clust (strict)"("Visible"=TRUE) -> ()  [unwired: 2 in, 2 out]
        n205 = property on="Motor" class="Clust (strict)"("Visible"=w334) -> ()  [unwired: 2 in, 2 out]
        n206 = property on="Slider" class="Slide (strict)"("Visible"=w334) -> ()  [unwired: 2 in, 2 out]
        n207 = property on="On/Off" class="Bool (strict)"("Visible"=w334) -> ()  [unwired: 2 in, 2 out]
        n208 = property on="Rev/Fwd" class="Clust (strict)"("Visible"=w334) -> ()  [unwired: 2 in, 2 out]
        n209 = property on="Ring" class="Ring (strict)"("Visible"=w334) -> ()  [unwired: 2 in, 2 out]
      }
      event "Listbox": Double Click {
        n210 = event-data() -> ("PlatMods.Shift"=w342:bool, "Row"=w344:i32)  [unwired: 1 in]
        n211 = case shown="False" w342 {
          tunnel: w344 -> [w348 _]
          tunnel: 1 -> [w347 _]
          frame False {
            n212 = property on="Listbox" class="LstBox (strict)"() -> ("Item Symbols"=w346:i32[])  [unwired: 2 in, 2 out]
            n213 = Replace Array Subset(array=w346, new element=w347, index=w348) -> (w345:i32[])
            n214 = property on="Listbox" class="LstBox (strict)"("Item Symbols"=w345) -> ()  [unwired: 2 in, 2 out]
          }
          frame True {
            w349 = 0 ("Top Row")
            n215 = property on="Listbox" class="LstBox (strict)"() -> ("Number of Rows"=w351:u32)  [unwired: 2 in, 2 out]
            n216 = Initialize Array(0, w351) -> (w350:i32[])
            n217 = property on="Listbox" class="LstBox (strict)"("Top Row"=w349, "Value"=w349, "Item Symbols"=w350) -> ()  [unwired: 2 in, 2 out]
          }
        }
      }
      event "Listbox": Key Down {
        n218 = event-data() -> ("VKey"=w355:T13)  [unwired: 1 in]
        n219 = case shown="\"Left\", \"Right\"" w355 {
          selector: w355 -> [w360 _]
          tunnel: eventvkey."Left" ("VKey") -> [w358 _]
          frame "Left", "Right" {
            n220 = Equal?(x=w358, y=w360) -> (x = y?=w359:bool)
            n221 = Select(t=0, s=w359, f=1) -> (s? t:f=w361:i32)
            n222 = property on="Listbox" class="LstBox (strict)"() -> ("Item Symbols"=w364:i32[])  [unwired: 2 in, 2 out]
            n223 = Replace Array Subset(array=w364, new element=w361, index="Listbox") -> (w363:i32[])
            n224 = property on="Listbox" class="LstBox (strict)"("Item Symbols"=w363) -> ()  [unwired: 2 in, 2 out]
          }
          frame Default {
          }
        }
      }
      event "DB Camera Config": Value Change {
        n225 = event-data() -> ("NewVal"=w368:bool)  [unwired: 1 in]
        n226 = case shown="False" w368 {
          tunnel: w367 -> [w377 _]
          tunnel: [w370 w388] -> w366
          tunnel: w365 -> [w369 w388]
          frame False {
            w384 = "Camera"
            w387 = FALSE ("Visible")
            n227 = local read "Camera Settings"() -> (w376:T3)
            n228 = Index Array(array=w377) -> (element=w380:cluster{string[]})  [unwired: 1 in]
            n229 = Unbundle(w376) -> ("Frate Rate"=w375:i32, "Compression"=w374:i32, "Size"=w378:u16)
            n230 = Unbundle(w380) -> (w379:string[])
            n231 = Index Array(array=w379, index=w378) -> (element=w373:string)
            n232 = call-poly <vilib>:"Write Key.vi"("section"=w384, "value"=w373, "key"="Size", "refnum"=w369) -> ("refnum out"=w386:T12)  [unwired: 2 in, 5 out]
            n233 = call-poly <vilib>:"Write Key.vi"("section"=w384, "value"=w375, "key"="FrameRate", "refnum"=w386) -> ("refnum out"=w385:T12)  [unwired: 1 in, 6 out]
            n234 = property on="Camera Settings" class="Clust (strict)"("Visible"=w387) -> ()  [unwired: 2 in, 2 out]
            n235 = local write "DB Camera Config"(w387) -> ()
            n236 = call-poly <vilib>:"Write Key.vi"("section"=w384, "value"=w374, "key"="Compression", "refnum"=w385) -> ("refnum out"=w371:T12)  [unwired: 1 in, 6 out]
            n237 = call <vilib>:"Close Config Data.vi"("refnum"=w371) -> ("file path"=w372:path)  [unwired: 2 in, 8 out]
            n238 = call <vilib>:"Open Config Data.vi"("configuration file path"=w372) -> ("refnum"=w370:T12)  [unwired: 8 in, 2 out]
          }
          frame True {
            n239 = property on="Camera Settings" class="Clust (strict)"("Visible"=TRUE) -> ()  [unwired: 2 in, 2 out]
          }
        }
      }
      event "Camera Settings": Value Change {
        n240 = event-data() -> ("NewVal"=w401:T3)  [unwired: 1 in]
        n241 = Index Array(array=w397) -> (element=w396:cluster{string[]})  [unwired: 1 in]
        n242 = Unbundle(w401) -> ("Frate Rate"=w392:i32, "Compression"=w391:i32, "Size"=w394:u16)
        n243 = Unbundle(w396) -> (w395:string[])
        n244 = Index Array(array=w395, index=w394) -> (element=w393:string)
        n245 = Format Into String(format string="%s   %dfps   %d%%", w393, w392, w391) -> (resulting string=w398:string)  [unwired: 2 in, 1 out]
        n246 = Build Array(w398) -> (w399:string[])
        n247 = property on="DB Camera Config" class="Bool (strict)"("Strings [4]"=w399) -> ()  [unwired: 2 in, 2 out]
      }
      event "Motor.Enable": Value Change {
        n248 = event-data() -> ("NewVal"=w407:bool)  [unwired: 1 in]
        n249 = Unbundle("Motor") -> ("Value"=w406:dbl)  [unwired: 1 out]
        n250 = Select(t=w406, s=w407, f=0.0) -> (s? t:f=w404:dbl)
        n251 = call <vilib>:"NT Write Number.vi"("Numeric"=w404, "Name"=w403) -> ()  [unwired: 9 in, 1 out]
      }
      event "Slider": Value Change {
        n252 = event-data() -> ("NewVal"=w410:dbl)  [unwired: 1 in]
        n253 = call <vilib>:"NT Write Number.vi"("Numeric"=w410, "Name"=w411) -> ()  [unwired: 9 in, 1 out]
      }
      event "On/Off": Value Change {
        n254 = event-data() -> ("NewVal"=w415:bool)  [unwired: 1 in]
        n255 = Boolean To (0,1)(Boolean=w415) -> (0, 1=w414:i16)
        n256 = call <vilib>:"NT Write Number.vi"("Numeric"=w414, "Name"=w413) -> ()  [unwired: 9 in, 1 out]
      }
      event "Rev/Fwd": Value Change {
        n257 = event-data() -> ("NewVal.Forward"=w423:bool, "NewVal.Reverse"=w422:bool)  [unwired: 1 in]
        n258 = Boolean To (0,1)(Boolean=w423) -> (0, 1=w419:i16)
        n259 = Boolean To (0,1)(Boolean=w422) -> (0, 1=w421:i16)
        n260 = Negate(x=w421) -> (-x=w420:i16)
        n261 = Add(x=w419, y=w420) -> (x+y=w418:i16)
        n262 = call <vilib>:"NT Write Number.vi"("Numeric"=w418, "Name"=w417) -> ()  [unwired: 9 in, 1 out]
      }
      event "Ring": Value Change {
        n263 = event-data() -> ("NewVal"=w427:u16)  [unwired: 1 in]
        n264 = property on="Ring" class="Ring (strict)"() -> ("Strings []"=w428:string[])  [unwired: 2 in, 2 out]
        n265 = Index Array(array=w428, index=w427) -> (element=w426:string)
        n266 = call <vilib>:"NT Write String.vi"("String"=w426, "Name"=w425) -> ()  [unwired: 9 in, 1 out]
      }
    }
  }
  n267 = Index Array(array=w13) -> (element=w14:cluster{string[]})  [unwired: 1 in]
  n268 = Unbundle(w14) -> (w12:string[])
  n269 = Match First String(2:w12, 3:w11) -> (0:w10:i32)  [unwired: 1 out]
  n270 = Bundle("value"=w16, "value"=w15, "index"=w10) -> (w4:cluster{"value":i32, "value":i32, "index":i32})  [unwired: 1 out]
  n271 = property on="On/Off" class="Bool (strict)"("Visible"=w27) -> ()  [unwired: 2 in, 2 out]
  n272 = property on="Motor" class="Clust (strict)"("Visible"=w27) -> ()  [unwired: 2 in, 2 out]
  n273 = property on="Progress" class="Clust (strict)"("Visible"=w27) -> ()  [unwired: 2 in, 2 out]
  n274 = property on="Ring" class="Ring (strict)"("Visible"=w27) -> ()  [unwired: 2 in, 2 out]
  n275 = property on="Camera Settings" class="Clust (strict)"("Val(Sgnl)"=w4) -> ()  [unwired: 2 in, 2 out]
  n276 = property on="Rev/Fwd" class="Clust (strict)"("Visible"=w27) -> ()  [unwired: 2 in, 2 out]
  n277 = property on="Camera Settings" class="Clust (strict)"("Visible"=w27) -> ()  [unwired: 2 in, 2 out]
  n278 = local write "DB Camera Config"(w27) -> ()
